vi "U3 Pin Configuration.vi"(1 "Timer/Counter Pin Offset":u8=4, 4 "Enable Counter1":bool, 6 "Enable Counter0":bool, 7 "FIO/EIO Analog Enable":i32, 8 "error in":errorcluster, 9 "Enable DAC1":bool, 10 "Number of Timers Enabled":u8, 11 "Handle In":i32) -> (0 "error out":errorcluster, 3 "Handle Out":i32)   [LabVIEW 2021]
panel:
  # "0 = All digital\n1= FIO0 analog\n65535 = All analog"
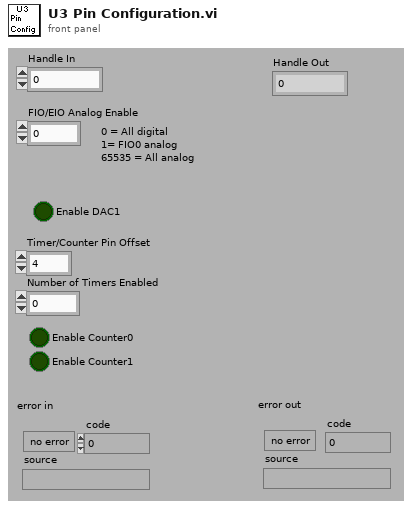
[diagram p1: front panel]
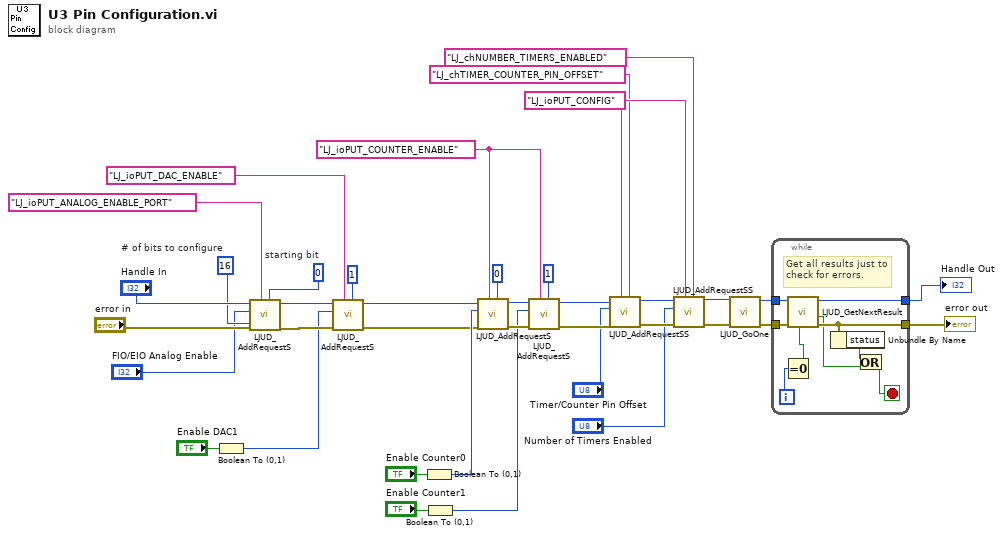
[diagram p0: block diagram]
diagram:
  w2 = 16  # # of bits to configure
  w25 = 0  # starting bit
  w22 = "LJ_ioPUT_COUNTER_ENABLE" ("Channel")
  w32 = "LJ_ioPUT_CONFIG" ("IOType")
  n1 = Boolean To (0,1)(Boolean="Enable DAC1") -> (0, 1=w6:i16)
  n2 = call "LJUD_AddRequestS.vi"("Channel"=w25, "x1"=w2, "IOType"="LJ_ioPUT_ANALOG_ENABLE_PORT" ("Channel"), "error in"="error in", "Value"="FIO/EIO Analog Enable", "Handle In"="Handle In") -> ("error out"=w10:errorcluster, "Handle Out"=w11:i32)  [unwired: 4 in]
  n3 = call "LJUD_AddRequestS.vi"("Channel"=1, "IOType"="LJ_ioPUT_DAC_ENABLE" ("Channel"), "error in"=w10, "Value"=w6, "Handle In"=w11) -> ("error out"=w9:errorcluster, "Handle Out"=w8:i32)  [unwired: 5 in]
  n4 = Boolean To (0,1)(Boolean="Enable Counter0") -> (0, 1=w15:i16)
  n5 = Boolean To (0,1)(Boolean="Enable Counter1") -> (0, 1=w14:i16)
  n6 = call "LJUD_AddRequestS.vi"("Channel"=0, "IOType"=w22, "error in"=w9, "Value"=w15, "Handle In"=w8) -> ("error out"=w27:errorcluster, "Handle Out"=w26:i32)  [unwired: 5 in]
  n7 = call "LJUD_AddRequestS.vi"("Channel"=1, "IOType"=w22, "error in"=w27, "Value"=w14, "Handle In"=w26) -> ("error out"=w24:errorcluster, "Handle Out"=w23:i32)  [unwired: 5 in]
  n8 = call "LJUD_AddRequestSS.vi"("Channel"="LJ_chTIMER_COUNTER_PIN_OFFSET", "IOType"=w32, "error in"=w24, "Value"="Timer/Counter Pin Offset", "Handle In"=w23) -> ("error out"=w37:errorcluster, "Handle Out"=w38:i32)  [unwired: 5 in]
  n9 = call "LJUD_AddRequestSS.vi"("Channel"="LJ_chNUMBER_TIMERS_ENABLED", "IOType"=w32, "error in"=w37, "Value"="Number of Timers Enabled", "Handle In"=w38) -> ("error out"=w36:errorcluster, "Handle Out"=w35:i32)  [unwired: 5 in]
  n10 = call "LJUD_GoOne.vi"("error in"=w36, "Handle In"=w35) -> ("error out"=w34:errorcluster, "Handle Out"=w33:i32)  [unwired: 8 in]
  n11 = while {
    tunnel: [w41] -> w16
    tunnel: [w43] -> w29
    tunnel: w33 -> [w44]
    tunnel: w34 -> [w45]
    i -> [w40]
    stop <- w47 stop-if-true
    # "Get all results just to\ncheck for errors."
    n12 = Equal To 0?(x=w40) -> (x = 0?=w46:bool)
    n13 = call "LJUD_GetNextResult.vi"("GetFirst"=w46, "error in"=w45, "Handle In"=w44) -> ("error out"=w43:errorcluster, "LJE_NO_MORE_DATA_AVAILABLE"=w39:bool, "Handle Out"=w41:i32)  [unwired: 3 in, 3 out]
    n14 = Unbundle By Name(w43) -> ("status"=w42:bool)
    n15 = Or(x=w42, y=w39) -> (x .or. y?=w47:bool)
  }
  "error out" <- w29
  "Handle Out" <- w16
